vi "TSPopup.Demo.vi"() -> ()   [LabVIEW 2013]
doc: "Demo for Type Sensitive Popup\n\nType Sensitive Popup \nCopyright © 2007, J. David Saunders\nAll rights reserved."
uses:
  TSPopup.Popup Cluster.ctl
  TSPopup.Grid.Cell Info.ctl
  TSPopup.Data Type.ctl
panel:
  in  "Popups":T1 {"Boolean" items=["False", "True"]; "Ring" items=["Shake", "Bake", "Blend", "Liquify", "Obliterate"]}
  in  "Cell Info (type only)":T2
  in  "stop":bool
  in  "Tests to Run":i32(listbox)
  in  "Signal Settings":i32(listbox)
  # "Run.   Click on the different cells to see \na few different data selection possibilities."
  # "Allowed controls :\n\nTable\nListbox\nMulticolumn Listbox\nTree\nString (why not?)"
  # "Data Types Implemented:\n\nNo Popup           Ring\nString                 Captioned String\nInteger              Captioned Integer\nFloat                  Button Color\nColor                  2 Integer Cluster\nBoolean             4 Integer Cluster"
  # "Type Sensitive\nPopup"
  # "Boolean Colors"
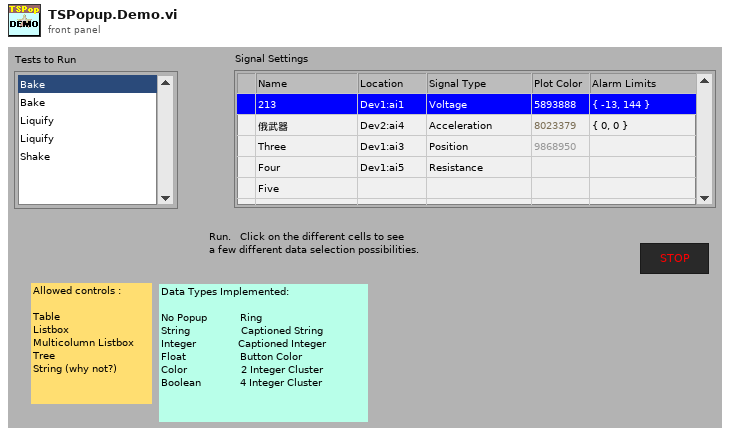
[diagram p1: front panel]
types:
  T1 = typedef "TSPopup.Popup Cluster.ctl" = cluster{"Unknown":bool, "Unknown 2":bool, "String":string, "Integer":i32, "Float":dbl, "Color":u32, "Boolean":u32, "Ring":u32, "Captioned String":cluster{"String":string, "OK":bool, "Cancel":bool}, "Captioned Integer":cluster{"First":i32, "OK":bool, "Cancel":bool}, "Boolean Colors":cluster{"False":cluster{"FG":u32, "BG":u32}, "True":cluster{"FG":u32, "BG":u32}, "T  to  F":cluster{"FG":u32, "BG":u32}, "F  to  T":cluster{"FG":u32, "BG":u32}, "OK":bool, "Cancel":bool}, "2-Int Cluster":cluster{"First":i32, "Second":i32, "OK":bool, "Cancel":bool}, "4-Int Cluster":cluster{"First":i32, "Second":i32, "Third":i32, "Fourth":i32, "OK":bool, "Cancel":bool}}
  T2 = typedef "TSPopup.Grid.Cell Info.ctl" = cluster{"Tag":string, "Row":i32, "Column":i32, "In Symbol?":bool, "In Data?":bool, "Cell String":string, "Ctl Refnum":refnum<vi>, "Prop Type":T3, "Ring Strings":string[]}
  T3 = typedef "TSPopup.Data Type.ctl" = enum16{"Unkown", "NO POPUP", "String", "Integer", "Float", "Color", "Boolean", "Ring", "Captioned String", "Captioned Integer", "Button Color", "2 Int Cluster", "4 Int Cluster"}
  T4 = typedef "LVPoint32TypeDef.ctl" = cluster{"Horizontal":i32, "Vertical":i32}
  T5 = typedef "TSPopup.Popup Call Parameters.ctl" = cluster{"Prop Type":T3, "Initial Value":variant, "Caption Strings":string[], "Ring Strings":string[], "Cell Rect":cluster{"left":i16, "top":i16, "right":i16, "bottom":i16}, "Mouse Coords":cluster{"x":i16, "y":i16}, "Call Data":variant}
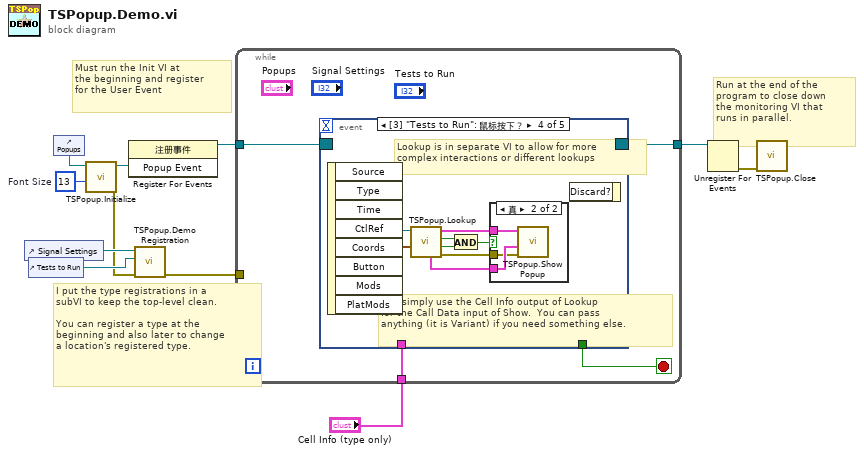
[diagram p0: block diagram]
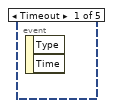
[diagram p2: hidden frame]
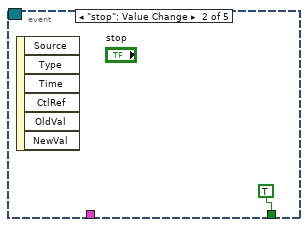
[diagram p3: hidden frame]
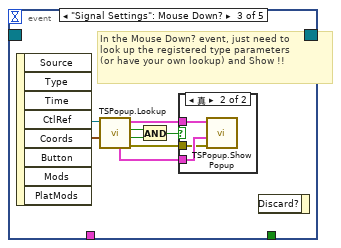
[diagram p4: hidden frame]
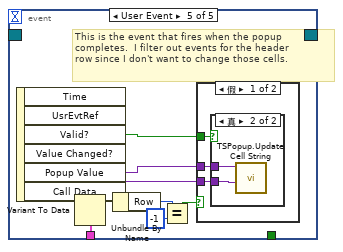
[diagram p7: hidden frame]
diagram:
  w10 = u32 13  # Font Size
  # "Run at the end of the\nprogram to close down\nthe monitoring VI that\nruns in parallel."
  # "I put the type registrations in a \nsubVI to keep the top-level clean.\n\nYou can register a type at the\nbeginning and also later to change\na location's registered type."
  # "Must run the Init VI at\nthe beginning and register\nfor the User Event"
  n1 = control-ref of="Signal Settings"() -> (w5:refnum<vi>)
  n2 = control-ref of="Tests to Run"() -> (w4:refnum<vi>)
  n3 = control-ref of="Popups"() -> (w11:refnum<vi>)
  n4 = call "TSPopup.Initialize.vi"("Font Size"=w10, "Popup Cluster Ref"=w11) -> ("error out"=w1:errorcluster, "Popup Event"=w9:refnum<user-event>)  [unwired: 8 in]
  n5 = register-events(w9) -> (reference out=w8:refnum<event-registration>)  [unwired: 2 in, 1 out]
  n6 = call "TSPopup.Demo Registration.vi"("error in (no error)"=w1, "Tests to Run ref"=w4, "Signal Settings ref"=w5) -> ("error out"=w2:errorcluster)  [unwired: 8 in]
  n7 = while {
    tunnel: w8 -> [w15]
    tunnel: [w14] -> w7
    tunnel: w2 -> [_]
    tunnel: "Cell Info (type only)" -> [w12]
    stop <- w13 stop-if-true
    n8 = event shown="[3] \"Tests to Run\": 鼠标按下？" {
      selector: w15 -> [_ _ _ _ _]
      dyn-events: [_ _ _ _ _] -> w14
      timeout: _ -> [_ _ _ _ _]
      tunnel: [_ TRUE _ _ _] -> w13
      tunnel: w12 -> [_ _ _ _ w43]
      event Timeout {
        n9 = event-data() -> ()  [unwired: 1 in, 2 out]
      }
      event "stop": Value Change {
        n10 = event-data() -> ()  [unwired: 1 in, 6 out]
      }
      event "Signal Settings": Mouse Down? {
        # "In the Mouse Down? event, just need to\nlook up the registered type parameters\n(or have your own lookup) and Show !!"
        n11 = event-data() -> ("CtlRef"=w24:refnum<vi>, "Coords"=w23:T4)  [unwired: 1 in, 6 out]
        n12 = call "TSPopup.Lookup.vi"("Point"=w23, "Ctl Refnum"=w24) -> ("error out"=w17:errorcluster, "In Bounds?"=w21:bool, "Found"=w22:bool, "Popup Parameters"=w19:T5, "Cell Info (Call data)"=w18:T2)  [unwired: 5 in]
        n13 = And(x=w22, y=w21) -> (x .and. y?=w20:bool)
        n14 = case shown="真" w20 {
          tunnel: w19 -> [_ w27]
          tunnel: w18 -> [_ w26]
          tunnel: w17 -> [_ w25]
          frame False {
          }
          frame True {
            n15 = call "TSPopup.Show Popup.vi"("error in (no error)"=w25, "Call Data (ignore if empty)"=w26, "Popup Parameters"=w27) -> ()  [unwired: 8 in, 1 out]
          }
        }
        n16 = event-data() -> ()  [unwired: 2 in, 1 out]
      }
      event "Tests to Run": Mouse Down? {
        # "Can simply use the Cell Info output of Lookup\nfor the Call Data input of Show.  You can pass\nanything (it is Variant) if you need something else."
        # "Lookup is in separate VI to allow for more\ncomplex interactions or different lookups"
        n17 = event-data() -> ("CtlRef"=w35:refnum<vi>, "Coords"=w34:T4)  [unwired: 1 in, 6 out]
        n18 = call "TSPopup.Lookup.vi"("Point"=w34, "Ctl Refnum"=w35) -> ("error out"=w28:errorcluster, "In Bounds?"=w32:bool, "Found"=w33:bool, "Popup Parameters"=w30:T5, "Cell Info (Call data)"=w29:T2)  [unwired: 5 in]
        n19 = And(x=w33, y=w32) -> (x .and. y?=w31:bool)
        n20 = case shown="真" w31 {
          tunnel: w30 -> [_ w38]
          tunnel: w29 -> [_ w37]
          tunnel: w28 -> [_ w36]
          frame False {
          }
          frame True {
            n21 = call "TSPopup.Show Popup.vi"("error in (no error)"=w36, "Call Data (ignore if empty)"=w37, "Popup Parameters"=w38) -> ()  [unwired: 8 in, 1 out]
          }
        }
        n22 = event-data() -> ()  [unwired: 2 in, 1 out]
      }
      event User Event {
        # "This is the event that fires when the popup\ncompletes.  I filter out events for the header\nrow since I don't want to change those cells."
        n23 = event-data() -> ("Valid?"=w46:bool, "Popup Value"=w45:variant, "Call Data"=w44:variant)  [unwired: 1 in, 3 out]
        n24 = Variant To Data(type=w43, Variant=w44) -> (data=w42:T2)  [unwired: 1 in, 1 out]
        n25 = Unbundle By Name(w42) -> ("Row"=w41:i32)
        n26 = Equal?(x=w41, y=-1) -> (x = y?=w39:bool)
        n27 = case shown="假" w39 {
          tunnel: w46 -> [w49 _]
          tunnel: w45 -> [w48 _]
          tunnel: w44 -> [w47 _]
          frame False {
            n28 = case shown="真" w49 {
              tunnel: w48 -> [_ w50]
              tunnel: w47 -> [_ w51]
              frame False {
              }
              frame True {
                n29 = call "TSPopup.Update Cell String.vi"("Call Data (must be Cell Info cluster)"=w51, "Popup Value"=w50) -> ()  [unwired: 9 in, 1 out]
              }
            }
          }
          frame True {
          }
        }
      }
    }
  }
  n30 = Unregister For Events(event registration refnum=w7) -> (error out=w6:errorcluster)  [unwired: 1 in]
  n31 = call "TSPopup.Close.vi"("error in (no error)"=w6) -> ()  [unwired: 10 in, 1 out]
